vi "SetPingAddresses.vi"(11 "Addresses to Ping(in)":T1) -> (3 "Addresses to Ping(out)":T1)   [LabVIEW 2011]
uses:
  Controls/PingElements.ctl
panel:
  in  "Addresses to Ping set":T1
  in  "Cancel Button":bool
  in  "OK Button":bool
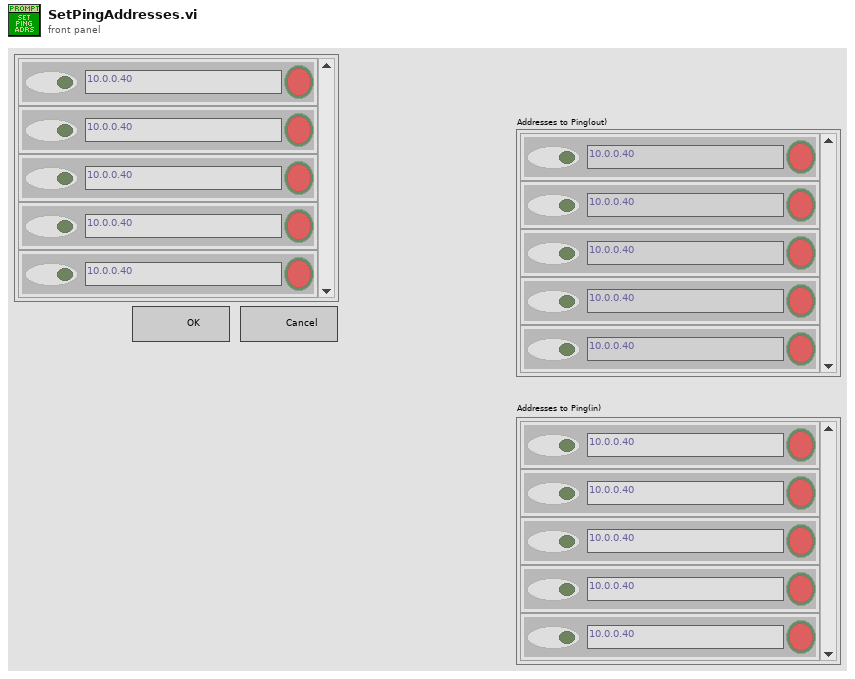
[diagram p1: front panel]
types:
  T1 = typedef "PingElements.ctl" = cluster{"AddressNode 1":string, "Response 1":bool, "Ping on Address 1":bool}[]
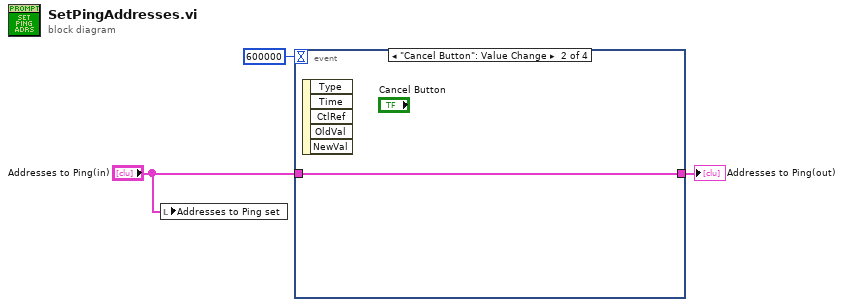
[diagram p0: block diagram]
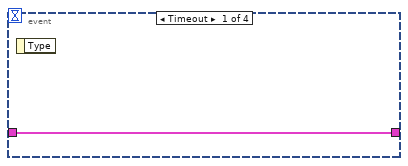
[diagram p2: hidden frame]
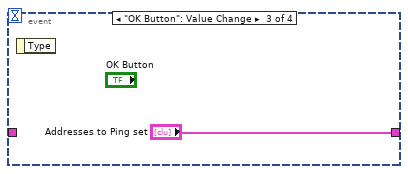
[diagram p3: hidden frame]
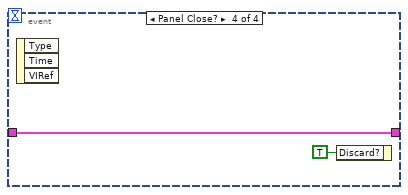
[diagram p4: hidden frame]
diagram:
  n1 = local write "Addresses to Ping set"("Addresses to Ping(in)") -> ()
  n2 = event shown="[1] \"Cancel Button\": Value Change" {
    selector: _ -> [_ _ _ _]
    dyn-events: _ -> [_ _ _ _]
    timeout: 600000 -> [_ _ _ _]
    tunnel: "Addresses to Ping(in)" -> [w4 w5 _ w7]
    tunnel: [w4 w5 "Addresses to Ping set" w7] -> w2
    event Timeout {
      n3 = event-data() -> ()  [unwired: 1 in, 1 out]
    }
    event "Cancel Button": Value Change {
      n4 = event-data() -> ()  [unwired: 1 in, 5 out]
    }
    event "OK Button": Value Change {
      n5 = event-data() -> ()  [unwired: 1 in, 1 out]
    }
    event Panel Close? {
      n6 = event-data() -> ()  [unwired: 1 in, 3 out]
      n7 = event-data("Discard?"=TRUE) -> ()  [unwired: 1 in, 1 out]
    }
  }
  "Addresses to Ping(out)" <- w2
